vi "Esempio scrittura su file.vi"() -> ()   [LabVIEW 2019]
uses:
  <vilib>/Utility/file.llb/Write Delimited Spreadsheet (string).vi
panel:
  out "Array String":string[][](array[string])
  in  "PPS":dbl=50.0
  in  "format string M3":string="%8.4f"
  in  "format string M2":string="%8.5f"
  in  "format string M1":string="%6.3f"
  in  "Time Stamp":timestamp=timestamp(3658819604.92083 s since 1904-01-01)
  in  "Frequenza":dbl[](array[numeric])=[7.0, 8.0, 9.0]
  in  "Fase":dbl[](array[numeric])=[4.0, 5.0, 6.0]
  in  "Ampiezza":dbl[](array[numeric])=[1.0, 2.0, 3.0]
  out "error out":errorcluster
  in  "Header":string[][](array[string])=[["Timestamp", "Ampiezza", "Fase", "Frequenza"], ["", "[V]", "[rad]", "[Hz]"]]
  in  "Nome File":string="file"
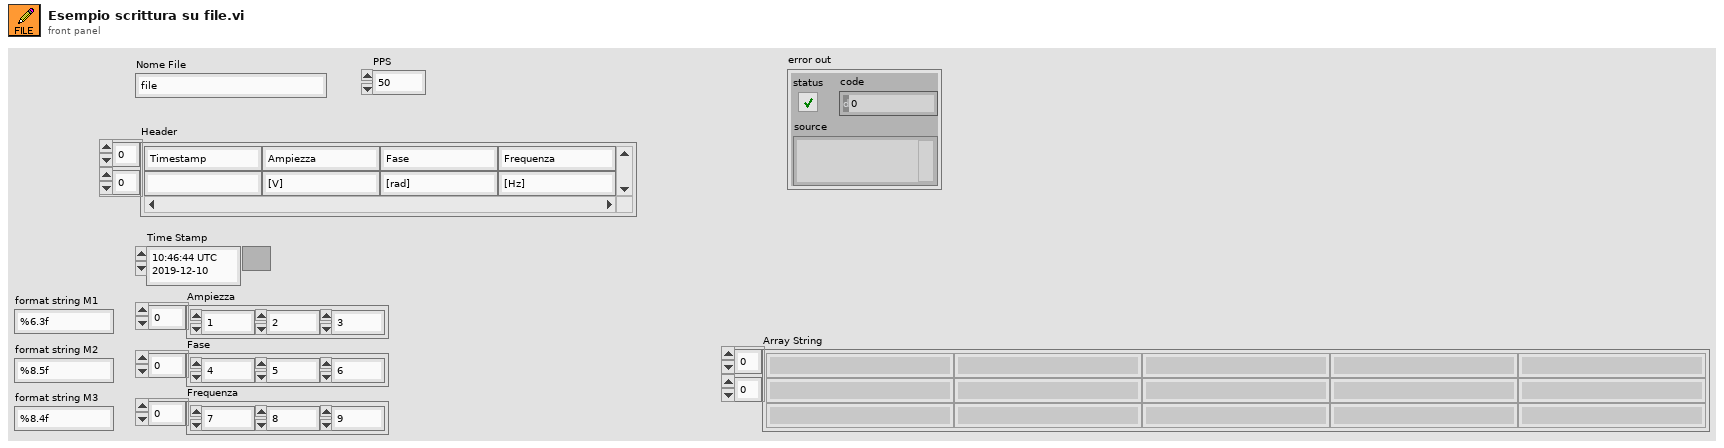
[diagram p1: front panel]
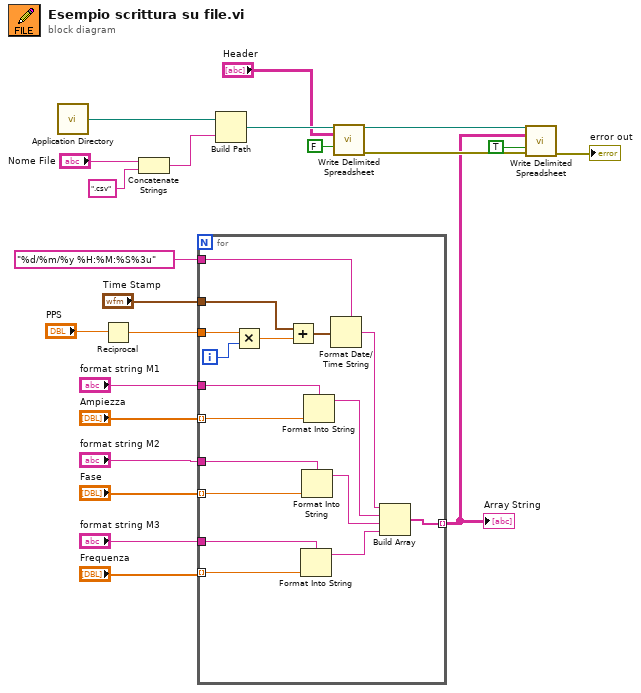
[diagram p0: block diagram]
diagram:
  n1 = call <vilib>:"Application Directory.vi"() -> ("Application Directory"=w22:path)
  n2 = Reciprocal(x="PPS") -> (1/x=w4:dbl)
  n3 = Concatenate Strings("Nome File", ".csv" ("string")) -> (w19:string)
  n4 = for {
    tunnel: "Ampiezza" -> [w39] mode=indexing
    tunnel: "Fase" -> [w38] mode=indexing
    tunnel: "Frequenza" -> [w23] mode=indexing
    tunnel: "format string M1" -> [w37]
    tunnel: "format string M2" -> [w24]
    tunnel: "format string M3" -> [w36]
    tunnel: [w32] -> w1 mode=indexing
    tunnel: w4 -> [w30]
    tunnel: "Time Stamp" -> [w28]
    tunnel: "%d/%m/%y %H:%M:%S%3u" ("time format string (%c)") -> [w27]
    i -> [w31]
    n5 = Multiply(x=w30, y=w31) -> (x*y=w29:dbl)
    n6 = Add(x=w28, y=w29) -> (x+y=w26:timestamp)
    n7 = Format Into String(format string=w36, w23) -> (resulting string=w33:string)  [unwired: 2 in, 1 out]
    n8 = Format Into String(format string=w24, w38) -> (resulting string=w34:string)  [unwired: 2 in, 1 out]
    n9 = Format Into String(format string=w37, w39) -> (resulting string=w35:string)  [unwired: 2 in, 1 out]
    n10 = Format Date/Time String(time format string (%c)=w27, seconds (now)=w26) -> (date/time string=w25:string)  [unwired: 1 in]
    n11 = Build Array(w25, w35, w34, w33) -> (w32:string[])
  }
  "Array String" <- w1
  n12 = Build Path(base path=w22, name or relative path=w19) -> (appended path=w18:path)
  n13 = call-poly <vilib>:"Write Delimited Spreadsheet.vi"("file path (dialog if empty)"=w18, "2D data"="Header", "append to file? (new file:F)"=FALSE) -> ("new file path (Not A Path if cancelled)"=w15:path, "error out"=w14:errorcluster)  [unwired: 11 in]
  n14 = call-poly <vilib>:"Write Delimited Spreadsheet.vi"("file path (dialog if empty)"=w15, "2D data"=w1, "append to file? (new file:F)"=TRUE, "error in (no error)"=w14) -> ("error out"=→"error out":errorcluster)  [unwired: 10 in, 1 out]
